vi "ueye get image size.vi"(8 "Error In":errorcluster, 11 ".NET (Reference)":refnum<k24>) -> (0 "Error Out":errorcluster, 1 "Height":i32, 2 "Width":i32, 3 ".NET (Reference)":refnum<k24>)   [LabVIEW 2017, in "Vision.lvlib"]
uses:
  Vision.lvlib
  C:/Users/Caleb/Desktop/nebraska-silicon-lab/pixel-gantry-extra/LV/bin/uEyeDotNet.dll
  bin/uEyeDotNet.dll
panel:
  out "SubSampFacVert":i32
  out "Subsampled Width":i32
  out "Binned Width":i32
  out "Subsampled Height":i32
  out "SubSampFacHor":i32
  out "Factored Width":i32
  out "Factored Height":i32
  out "Binned Height":i32
  out "Scaler":dbl
  out "BinFacVert":i32
  out "BinFaHor":i32
  out "bAbsPosY":bool
  out "bAbsPosX":bool
  out "Max Width":i32
  out "Max Height":i32
  out "s32PosY":i32
  out "s32PosX":i32
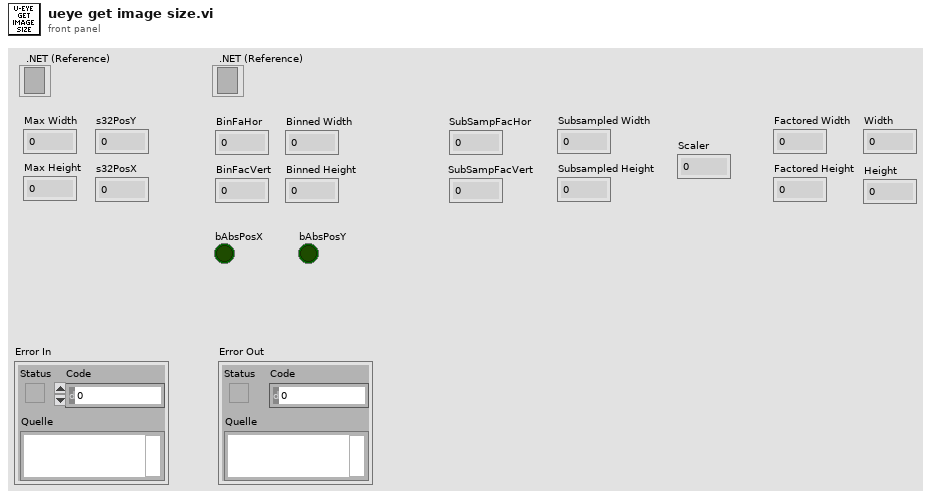
[diagram p1: front panel]
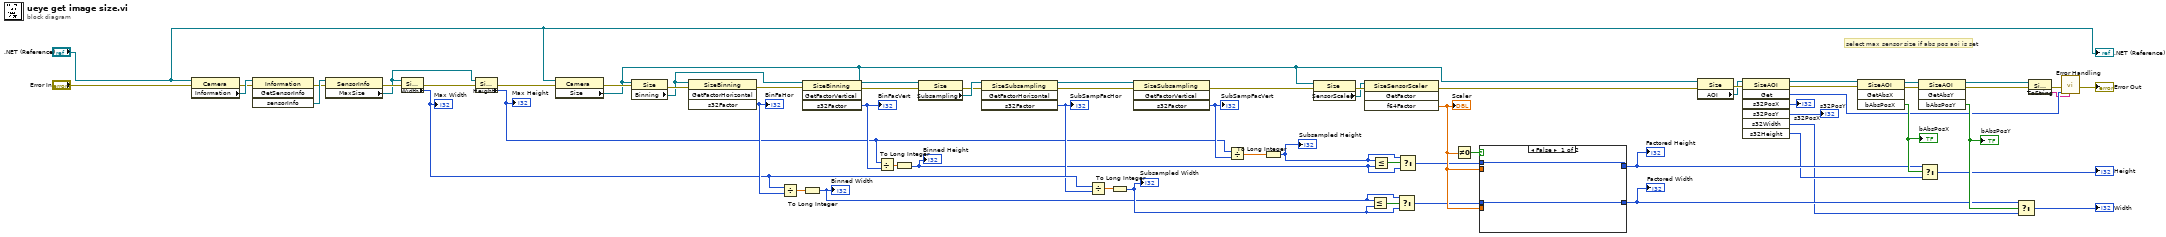
[diagram p0: block diagram]
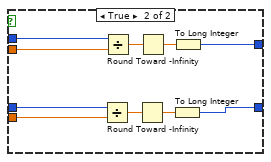
[diagram p2: hidden frame]
diagram:
  # "select max sensor size if abs pos aoi is set"
  n1 = property class="Camera"(reference=".NET (Reference)", error in="Error In") -> (error out=w62:errorcluster, "Information"=w64:refnum<k24>)  [unwired: 1 out]
  n2 = invoke class="Information" method="GetSensorInfo"(reference=w64, error in=w62) -> (error out=w61:errorcluster, "sensorInfo"=w63:refnum<k24>)  [unwired: 2 in, 2 out]
  n3 = property class="SensorInfo"(reference=w63, error in=w61) -> (error out=w60:errorcluster, "MaxSize"=w58:refnum<k24>)  [unwired: 1 out]
  n4 = property class="Size`1[[System.Int32, mscorlib,"(reference=w58, error in=w60) -> (error out=w59:errorcluster, "Width"=w22:i32)  [unwired: 1 out]
  "Max Width" <- w22
  n5 = property class="Size`1[[System.Int32, mscorlib,"(reference=w58, error in=w59) -> (error out=w57:errorcluster, "Height"=w19:i32)  [unwired: 1 out]
  "Max Height" <- w19
  n6 = property on="Eigenschaftsknoten" class="Camera"(reference=".NET (Reference)", error in=w57) -> (error out=w36:errorcluster, "Size"=w10:refnum<k24>)  [unwired: 1 out]
  n7 = property class="Size"(reference=w10, error in=w36) -> (error out=w46:errorcluster, "Binning"=w44:refnum<k24>)  [unwired: 1 out]
  n8 = invoke class="SizeBinning" method="GetFactorHorizontal"(reference=w44, error in=w46) -> (error out=w45:errorcluster, "s32Factor"=w23:i32)  [unwired: 2 in, 2 out]
  "BinFaHor" <- w23
  n9 = Divide(x=w22, y=w23) -> (x/y=w26:dbl)
  n10 = invoke class="SizeBinning" method="GetFactorVertical"(reference=w44, error in=w45) -> (error out=w31:errorcluster, "s32Factor"=w24:i32)  [unwired: 2 in, 2 out]
  "BinFacVert" <- w24
  n11 = To Long Integer(number=w26) -> (32bit integer=w13:i32)
  "Binned Width" <- w13
  n12 = Divide(x=w19, y=w24) -> (x/y=w41:dbl)
  n13 = To Long Integer(number=w41) -> (32bit integer=w16:i32)
  "Binned Height" <- w16
  n14 = property class="Size"(reference=w10, error in=w31) -> (error out=w32:errorcluster, "Subsampling"=w35:refnum<k24>)  [unwired: 1 out]
  n15 = invoke class="SizeSubsampling" method="GetFactorHorizontal"(reference=w35, error in=w32) -> (reference out=w33:refnum<k24>, error out=w34:errorcluster, "s32Factor"=w20:i32)  [unwired: 2 in, 1 out]
  "SubSampFacHor" <- w20
  n16 = Divide(x=w22, y=w20) -> (x/y=w25:dbl)
  n17 = To Long Integer(number=w25) -> (32bit integer=w14:i32)
  "Subsampled Width" <- w14
  n18 = invoke class="SizeSubsampling" method="GetFactorVertical"(reference=w33, error in=w34) -> (error out=w29:errorcluster, "s32Factor"=w21:i32)  [unwired: 2 in, 2 out]
  "SubSampFacVert" <- w21
  n19 = Divide(x=w19, y=w21) -> (x/y=w30:dbl)
  n20 = To Long Integer(number=w30) -> (32bit integer=w17:i32)
  "Subsampled Height" <- w17
  n21 = property class="Size"(reference=w10, error in=w29) -> (error out=w43:errorcluster, "SensorScaler"=w42:refnum<k24>)  [unwired: 1 out]
  n22 = invoke class="SizeSensorScaler" method="GetFactor"(reference=w42, error in=w43) -> (error out=w9:errorcluster, "f64Factor"=w28:dbl)  [unwired: 2 in, 2 out]
  "Scaler" <- w28
  n23 = Less Or Equal?(x=w13, y=w14) -> (x <= y?=w15:bool)
  n24 = Less Or Equal?(x=w17, y=w16) -> (x <= y?=w18:bool)
  n25 = Select(t=w13, s=w15, f=w14) -> (s? t:f=w11:i32)
  n26 = Select(t=w17, s=w18, f=w16) -> (s? t:f=w12:i32)
  n27 = Not Equal To 0?(x=w28) -> (x != 0?=w27:bool)
  n28 = case shown="False" w27 {
    tunnel: w12 -> [w68 w72]
    tunnel: w11 -> [w67 w70]
    tunnel: w28 -> [_ w71]
    tunnel: w28 -> [_ w69]
    tunnel: [w68 w74] -> w39
    tunnel: [w67 w73] -> w38
    frame False {
    }
    frame True {
      n29 = Divide(x=w70, y=w69) -> (x/y=w75:dbl)
      n30 = Divide(x=w72, y=w71) -> (x/y=w78:dbl)
      n31 = Round Toward -Infinity(1:w75) -> (0:w76:dbl)
      n32 = Round Toward -Infinity(1:w78) -> (0:w77:dbl)
      n33 = To Long Integer(number=w76) -> (32bit integer=w73:i32)
      n34 = To Long Integer(number=w77) -> (32bit integer=w74:i32)
    }
  }
  "Factored Height" <- w39
  "Factored Width" <- w38
  n35 = property class="Size"(reference=w10, error in=w9) -> (error out=w48:errorcluster, "AOI"=w47:refnum<k24>)  [unwired: 1 out]
  n36 = invoke class="SizeAOI" method="Get"(reference=w47, error in=w48) -> (reference out=w56:refnum<k24>, error out=w53:errorcluster, "Get"=w3:i32, "s32PosX"=→"s32PosX":i32, "s32PosY"=→"s32PosY":i32, "s32Width"=w5:i32, "s32Height"=w6:i32)  [unwired: 5 in]
  n37 = invoke class="SizeAOI" method="GetAbsX"(reference=w56, error in=w53) -> (reference out=w55:refnum<k24>, error out=w54:errorcluster, "bAbsPosX"=w50:bool)  [unwired: 2 in, 1 out]
  "bAbsPosX" <- w50
  n38 = invoke class="SizeAOI" method="GetAbsY"(reference=w55, error in=w54) -> (reference out=w52:refnum<k24>, error out=w51:errorcluster, "bAbsPosY"=w49:bool)  [unwired: 2 in, 1 out]
  "bAbsPosY" <- w49
  n39 = Select(t=w39, s=w50, f=w6) -> (s? t:f=→"Height":i32)
  n40 = Select(t=w38, s=w49, f=w5) -> (s? t:f=→"Width":i32)
  n41 = invoke class="SizeAOI" method="ToString"(reference=w52, error in=w51) -> (error out=w4:errorcluster, "ToString"=w2:string)  [unwired: 1 in, 1 out]
  n42 = call "Error Handling.vi"("Error String"=w2, "Error Code"=w3, "Error In"=w4) -> ("Error Out"=→"Error Out":errorcluster)  [unwired: 8 in]
  ".NET (Reference)" <- ".NET (Reference)"
